vi "Module Type.vi"(11 "Historian Module in":refnum<class "Historian Module.lvclass">) -> (2 "Module Type":string)   [LabVIEW 2020, in "VolatusHistorian.lvlib" / "Historian Module.lvclass"]
uses:
  Historian Module.lvclass
  Historian Module.lvclass/Historian Module.ctl
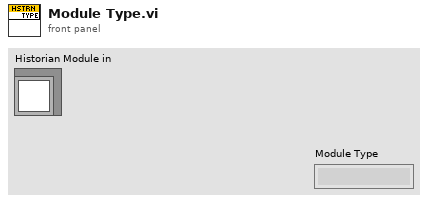
[diagram p1: front panel]
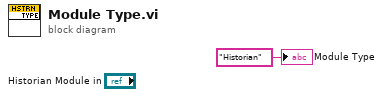
[diagram p0: block diagram]
diagram:
  "Module Type" <- "Historian" ("Module Type")
